vi "Read Data.vi"(8 "error in (no error)":errorcluster) -> (0 "error out":errorcluster, 3 "Normalized Data":dbl[][](array[numeric]), 5 "Character Images":picture[](array[picture]))   [LabVIEW 2018]
uses:
  <vilib>/Utility/file.llb/Read Delimited Spreadsheet (DBL).vi
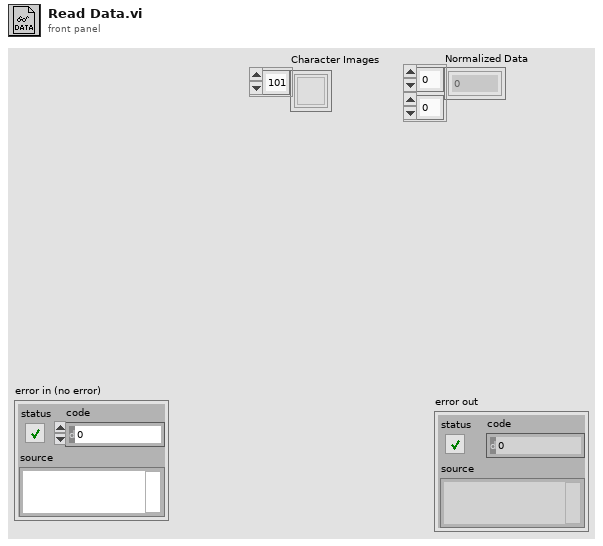
[diagram p1: front panel]
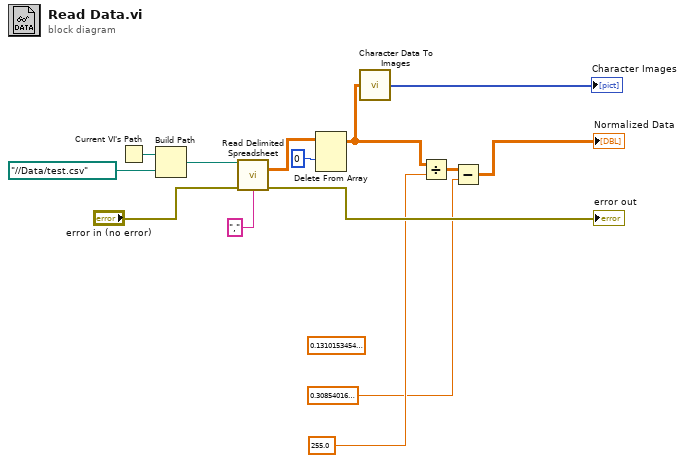
[diagram p0: block diagram]
diagram:
  (unwired) sgl 0.13101535 ("Mean")
  n1 = Current VI's Path() -> (path=w9:path)
  n2 = Build Path(base path=w9, name or relative path=path "../../Data/test.csv" ("path")) -> (appended path=w14:path)
  n3 = call-poly <vilib>:"Read Delimited Spreadsheet.vi"("file path (dialog if empty)"=w14, "error in (no error)"="error in (no error)", "delimiter (\\t)"="," ("delimiter (\\t)")) -> ("all rows"=w12:dbl[][], "error out"=→"error out":errorcluster)  [unwired: 7 in, 4 out]
  n4 = Delete From Array(array=w12, index (row)=0) -> (array with subset deleted=w2:dbl[][])  [unwired: 2 in, 1 out]
  n5 = call "Character Data To Images.vi"("All Rows of Data"=w2) -> ("Character Images"=→"Character Images":picture[])
  n6 = Divide(x=w2, y=sgl 255.0 ("Max")) -> (x/y=w5:dbl[][])
  n7 = Subtract(x=w5, y=sgl 0.30854017 ("standard deviation")) -> (x-y=→"Normalized Data":dbl[][])
